vi "Conductus Calibration Tables.vi"() -> ()   [LabVIEW 2024]
panel:
  in  "Voltage Bias":T1(ring)=enum."3 mV"
  in  "Sensor Type":T2(ring)=enum."Resistance1.0M "
  in  "stop":bool
  out "Excitation":string[](array[string])
  out "Scale Factor":dbl[](array[numeric]) format="%.2f"
  out "Units":enum16{"Logohms", "Ohms", "Volts"}[](array[ring])
  out "Type":string[](array[string])
  in  "delete":bool
  in  "add":bool
  in  "User Calibrations":i32[](listbox)
  out "Names":string[](array[string])
  in  "VISA session":refnum<visa-resource-name>
  # "Set Sensor Type and\nexcitation for curve to\nbe loaded, then press \"Add\""
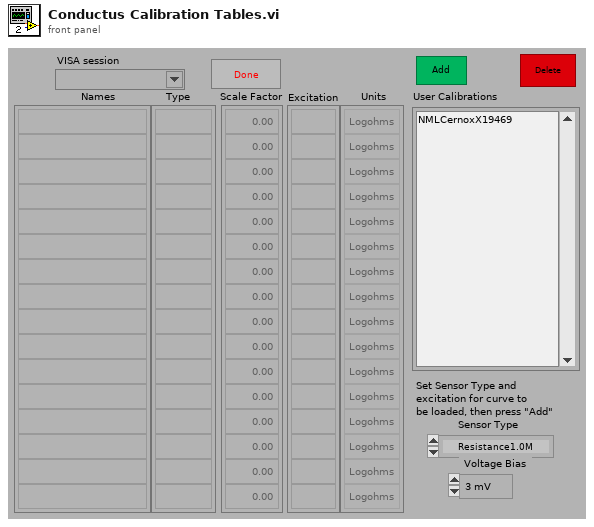
[diagram p1: front panel]
types:
  T1 = enum16{"10 mV", "3 mV", "1 mV", "320 uV", "100 uV", "32 uV", "10 uV"}
  T2 = enum16{"2V Diode", "6V Diode", "Platinum - 1 mA", "Platinum - 100µA", "Resistance1.0M "}
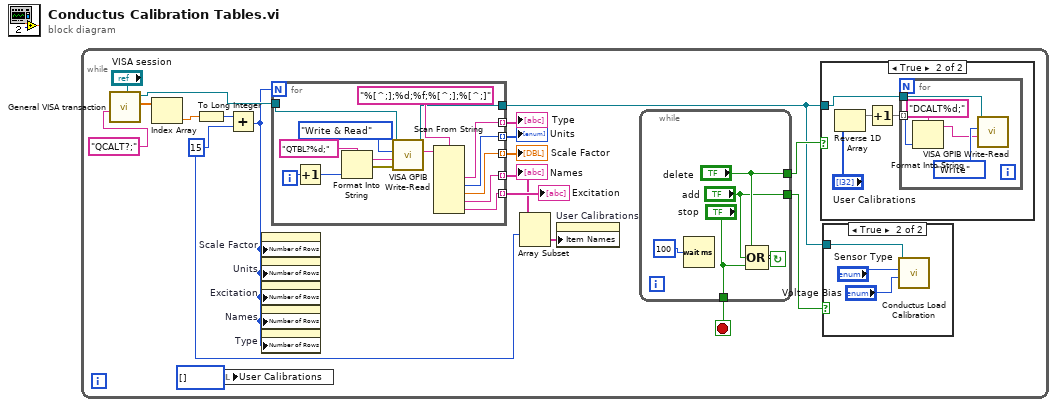
[diagram p0: block diagram]
diagram:
  n1 = while {
    stop <- w4 stop-if-true
    w2 = 15 ("y")
    n2 = call "General VISA transaction.vi"("Command String"="QCALT?;" ("String to Write"), "VISA Session"="VISA session") -> ("Measurement"=w17:dbl[], "dup VISA Session"=w16:refnum<visa-resource-name>)  [unwired: 4 in, 4 out]
    n3 = Index Array(array=w17) -> (element=w15:dbl)  [unwired: 1 in]
    n4 = To Long Integer(number=w15) -> (32bit integer=w14:i32)
    n5 = local write "User Calibrations"(i32[] [] ("User Calibrations")) -> ()
    n6 = Add(x=w14, y=w2) -> (x+y=w7:i32)
    n7 = property on="Scale Factor" class="Arr (strict)"("Number of Rows"=w7) -> ()  [unwired: 2 in, 2 out]
    n8 = property on="Units" class="Arr (strict)"("Number of Rows"=w7) -> ()  [unwired: 2 in, 2 out]
    n9 = property on="Excitation" class="Arr (strict)"("Number of Rows"=w7) -> ()  [unwired: 2 in, 2 out]
    n10 = property on="Names" class="Arr (strict)"("Number of Rows"=w7) -> ()  [unwired: 2 in, 2 out]
    n11 = property on="Type" class="Arr (strict)"("Number of Rows"=w7) -> ()  [unwired: 2 in, 2 out]
    n12 = for {
      N: w7 -> [_]
      tunnel: w16 -> [w45]
      tunnel: [w42] -> w8 mode=indexing
      tunnel: [w41] -> w13 mode=indexing
      tunnel: [w40] -> w12 mode=indexing
      tunnel: [w39] -> w11 mode=indexing
      tunnel: [w38] -> w10 mode=indexing
      tunnel: [w37] -> w1
      i -> [w51]
      n13 = Increment(x=w51) -> (x+1=w50:i32)
      n14 = Format Into String(format string="QTBL?%d;" ("Format String"), w50) -> (resulting string=w47:string, error out=w46:errorcluster)  [unwired: 2 in]
      n15 = call "VISA GPIB Write-Read.vi"("error in (no error)"=w46, "Command"=w47, "Action"=enum16{"Write", "Read", "Write & Read"}."Write & Read", "VISA resource name"=w45) -> ("String Returned"=w44:string, "dup VISA Session"=w37:refnum<visa-resource-name>)  [unwired: 4 in, 2 out]
      n16 = Scan From String(format string="%[^;];%d;%f;%[^;];%[^;]" ("Format String"), input string=w44) -> (output 1=w41:string, output 2=w40:i32, output 3=w39:dbl, output 4=w42:string, output 5=w38:string)  [unwired: 7 in, 3 out]
    }
    "Names" <- w8
    "Type" <- w13
    "Units" <- w12
    "Scale Factor" <- w11
    "Excitation" <- w10
    n17 = Array Subset(array=w8, index=w2) -> (w9:string[])  [unwired: 1 in]
    n18 = property on="User Calibrations" class="LstBox (strict)"("Item Names"=w9) -> ()  [unwired: 2 in, 2 out]
    n19 = while {
      tunnel: ["stop"] -> w4
      tunnel: ["add"] -> w5
      tunnel: ["delete"] -> w6
      stop <- w23 continue-if-true
      n20 = Wait (ms)(milliseconds to wait=u32 100) -> ()  [unwired: 1 out]
      n21 = Compound Arithmetic op=OR("delete", "add", "stop") -> (invert w23:bool)
    }
    n22 = case shown="True" w6 {
      tunnel: w1 -> [_ w29]
      frame False {
      }
      frame True {
        n23 = Reverse 1D Array(array="User Calibrations") -> (reversed array=w28:i32[])
        n24 = Increment(x=w28) -> (x+1=w31:i32[])
        n25 = for {
          tunnel: w31 -> [w35] mode=indexing
          tunnel: w29 -> [w34]
          n26 = Format Into String(format string="DCALT%d;" ("Format String"), w35) -> (resulting string=w32:string)  [unwired: 2 in, 1 out]
          n27 = call "VISA GPIB Write-Read.vi"("Command"=w32, "Action"=enum16{"Write", "Read", "Write & Read"}."Write", "VISA resource name"=w34) -> ()  [unwired: 5 in, 4 out]
        }
      }
    }
    n28 = case shown="True" w5 {
      tunnel: w1 -> [_ w25]
      frame False {
      }
      frame True {
        n29 = call "Conductus Load Calibration.vi"("Voltage Bias"="Voltage Bias", "Sensor Type"="Sensor Type", "Instrument Address"=w25) -> ()  [unwired: 3 in, 2 out]
      }
    }
  }
